vi "Perform_large_file_Analysis.vi"(0 "IntensityGraph in":refnum<vi>) -> (1 "Integral Spectrum":dbl[][](array[numeric]), 2 "size(s)":i32, 3 "Analysis_Data":T2, 4 "Spectrum Data":T1, 5 "Discr. Slope":cluster{"Array":dbl[], "Array":dbl[]})   [LabVIEW 2019]
uses:
  ESA_Data_Analysis_Global_VIs.vi
  <vilib>/Analysis/NI_AALPro.lvlib
panel:
  out "Ch#1 min peak index":i32
  out "Ch#2 min peak index":i32
  out "Ch#2 min peak":dbl
  out "Ch#1 min peak":dbl
  out "Waveform Graph":dbl[][](graph)
  out "Ch#2_Peak":dbl[](array[numeric])
  out "Ch#1_Peak":dbl[](array[numeric])
  out "channel name(s) out":string[](array[string])
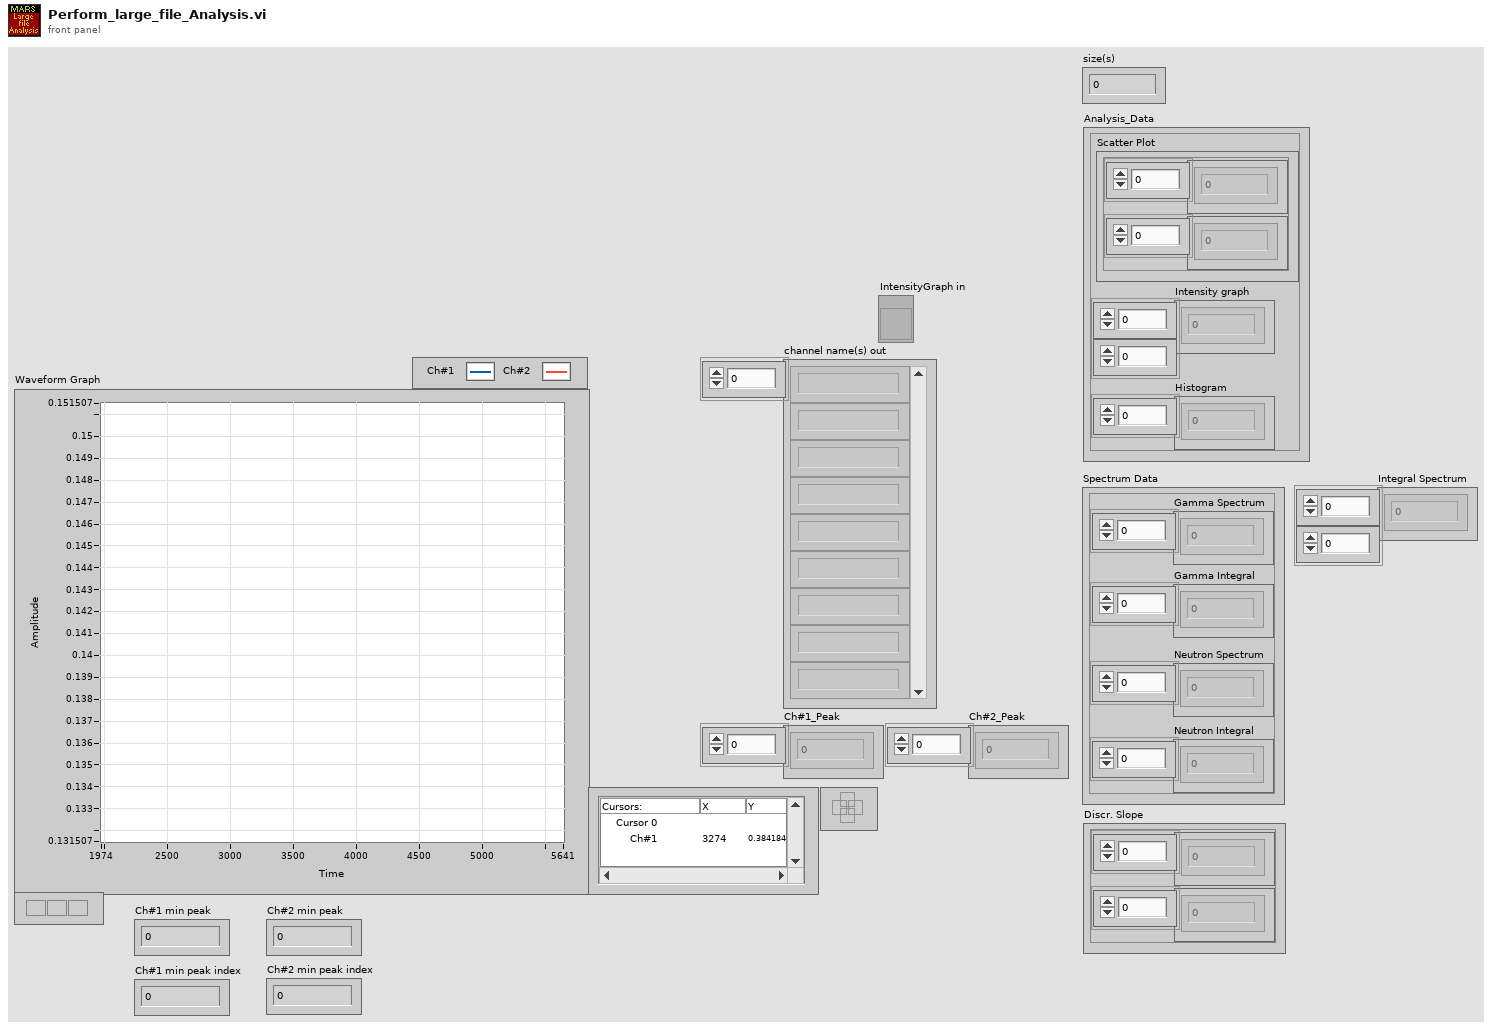
[diagram p1: front panel]
types:
  T1 = cluster{"Gamma Spectrum":dbl[], "Gamma Integral":dbl[], "Neutron Spectrum":dbl[], "Neutron Integral":dbl[]}
  T2 = cluster{"Scatter Plot":cluster{"Array":dbl[], "Array":dbl[]}, "Intensity graph":u32[][], "Histogram":u32[]}
  T3 = cluster{"Cursor.Cursor X1":dbl, "Cursor.Cursor Y1":dbl, "Cursor.Cursor X2":dbl, "Cursor.Cursor Y2":dbl}
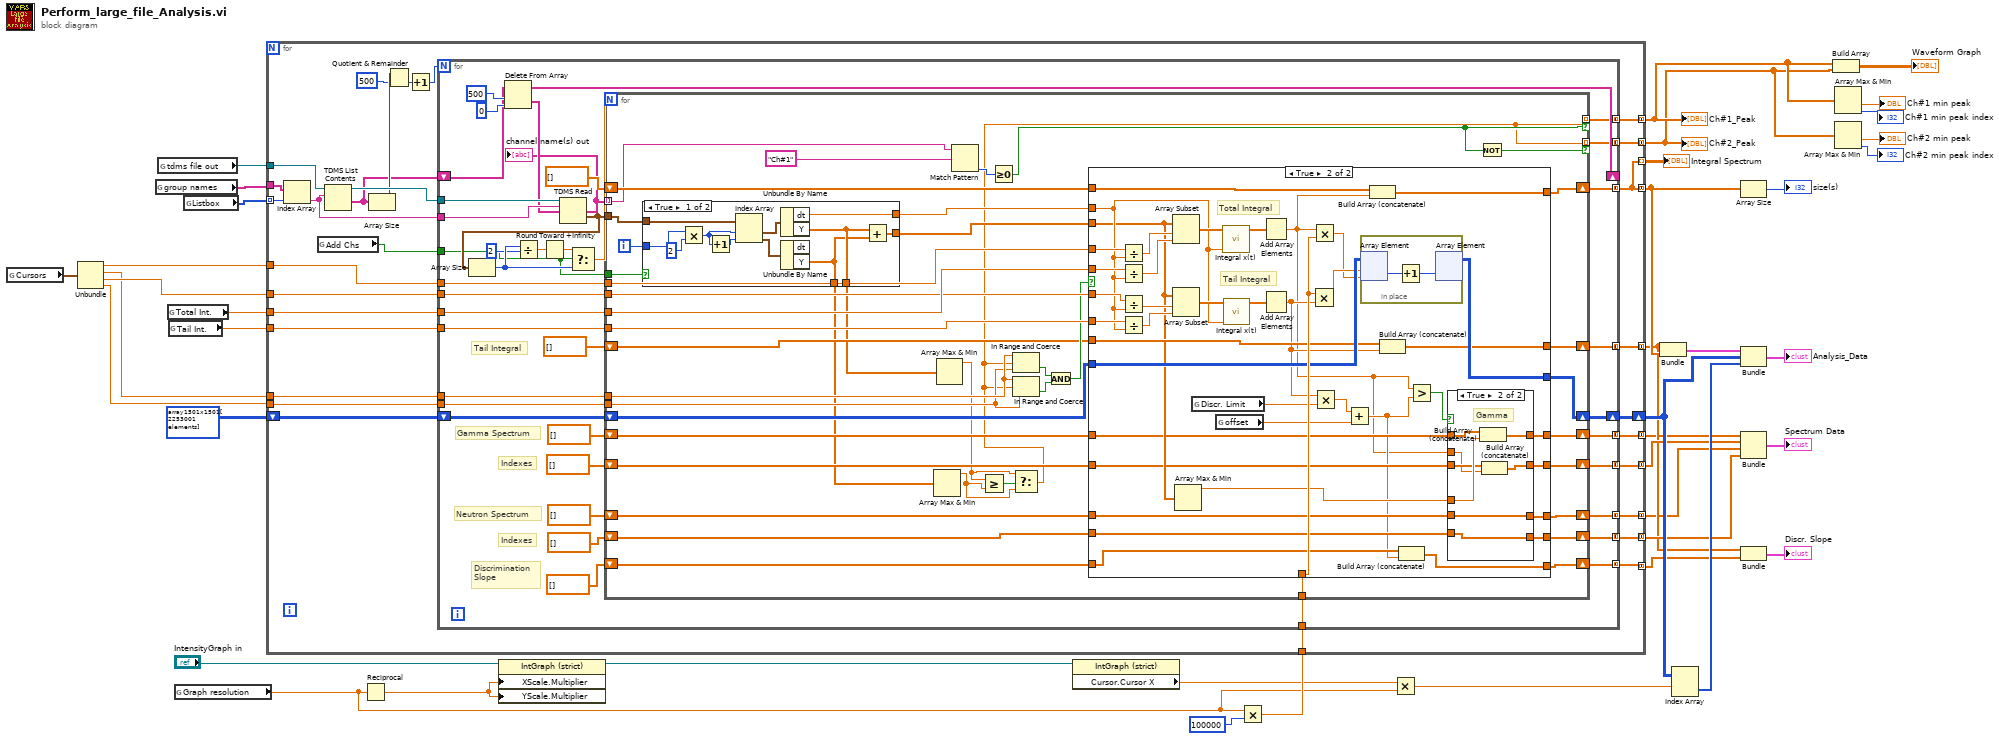
[diagram p0: block diagram]
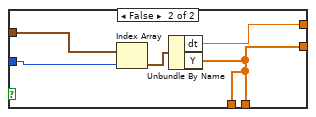
[diagram p2: hidden frame]
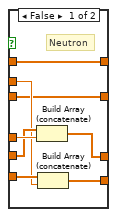
[diagram p4: hidden frame]
diagram:
  n1 = global read "ESA_Data_Analysis_Global_VIs.vi" "Cursors"() -> (w18:T3)
  n2 = Unbundle(w18) -> ("Cursor.Cursor X1"=w31:dbl, "Cursor.Cursor Y1"=w29:dbl, "Cursor.Cursor X2"=w30:dbl, "Cursor.Cursor Y2"=w28:dbl)
  n3 = global read "ESA_Data_Analysis_Global_VIs.vi" "group names"() -> (w20:string[])
  n4 = global read "ESA_Data_Analysis_Global_VIs.vi" "tdms file out"() -> (w21:refnum<k34>)
  n5 = global read "ESA_Data_Analysis_Global_VIs.vi" "Total Int."() -> (w24:dbl)
  n6 = global read "ESA_Data_Analysis_Global_VIs.vi" "Tail Int."() -> (w23:dbl)
  n7 = global read "ESA_Data_Analysis_Global_VIs.vi" "Graph resolution"() -> (w22:dbl)
  n8 = global read "ESA_Data_Analysis_Global_VIs.vi" "Listbox"() -> (w19:i32[])
  n9 = Reciprocal(x=w22) -> (1/x=w40:dbl)
  n10 = property on="Property Node" class="IntGraph (strict)"(reference="IntensityGraph in", "XScale.Multiplier"=w40, "YScale.Multiplier"=w40) -> (reference out=w36:refnum<vi>)  [unwired: 1 in, 1 out]
  n11 = property on="Property Node" class="IntGraph (strict)"(reference=w36) -> ("Cursor.Cursor X"=w35:dbl)  [unwired: 1 in, 2 out]
  n12 = Multiply(x=w22, y=100000) -> (x*y=w38:dbl)
  n13 = for {
    tunnel: w21 -> [w70]
    tunnel: w20 -> [w68]
    tunnel: w19 -> [w67] mode=indexing
    tunnel: w31 -> [w63]
    tunnel: w30 -> [w62]
    tunnel: w24 -> [w61]
    tunnel: w23 -> [w60]
    tunnel: w38 -> [w59]
    shift-right: [w57] -> w27
    shift-left: u32[][] array1501x1501[2253001 elements] -> [w58]
    tunnel: [w46] -> w33 mode=concatenating
    tunnel: [w56] -> w12 mode=concatenating
    tunnel: w29 -> [w53]
    tunnel: w28 -> [w52]
    tunnel: [w51] -> w9 mode=concatenating
    tunnel: [w50] -> w10 mode=concatenating
    tunnel: [w49] -> w17 mode=concatenating
    tunnel: [w48] -> w16 mode=concatenating
    tunnel: [w47] -> w13 mode=concatenating
    tunnel: [w46] -> w8 mode=indexing
    tunnel: [w44] -> w6 mode=concatenating
    tunnel: [w43] -> w5 mode=concatenating
    n14 = Index Array(array=w68, index=w67) -> (element=w64:string)
    n15 = global read "ESA_Data_Analysis_Global_VIs.vi" "Add Chs"() -> (w42:bool)
    n16 = TDMS List Contents(6:w64, 7:w70) -> (1:w55:string[], 3:w69:refnum<k34>)  [unwired: 1 in, 2 out]
    n17 = Array Size(array=w55) -> (size(s)=w66:i32)
    n18 = Quotient & Remainder(x=w66, y=500) -> (floor(x/y)=w54:i32)  [unwired: 1 out]
    n19 = Increment(x=w54) -> (x+1=w45:i32)
    n20 = for {
      N: w45 -> [_]
      tunnel: w69 -> [w110]
      tunnel: w64 -> [w100]
      tunnel: w63 -> [w109]
      tunnel: w62 -> [w108]
      tunnel: w61 -> [w107]
      tunnel: w60 -> [w106]
      tunnel: w59 -> [w105]
      shift-right: [w103] -> w57
      shift-left: w58 -> [w104]
      tunnel: [w102] -> w46 mode=concatenating
      tunnel: [w101] -> w56 mode=concatenating
      shift-right: [w96] -> _
      shift-left: w55 -> [w97]
      tunnel: w53 -> [w94]
      tunnel: w52 -> [w93]
      tunnel: [w88] -> w51 mode=concatenating
      tunnel: [w87] -> w50 mode=concatenating
      tunnel: [w85] -> w49 mode=concatenating
      tunnel: [w83] -> w48 mode=concatenating
      tunnel: [w81] -> w47 mode=concatenating
      tunnel: [w79] -> w44 mode=concatenating
      tunnel: [w78] -> w43 mode=concatenating
      tunnel: w42 -> [w71]
      # "Tail Integral"
      # "Discrimination\nSlope"
      # "Indexes"
      # "Indexes"
      # "Neutron Spectrum"
      # "Gamma Spectrum"
      n21 = Delete From Array(array=w97, length=500, index=0) -> (deleted portion=w95:string[], array with subset deleted=w96:string[])
      n22 = TDMS Read(0:w110, 5:w100, 7:w95) -> (8:w80:string[], 10:w77:waveform(dbl)[])  [unwired: 5 in, 4 out]
      "channel name(s) out" <- w80
      n23 = Array Size(array=w77) -> (size(s)=w76:i32)
      n24 = Divide(x=w76, y=2) -> (x/y=w73:dbl)
      n25 = Round Toward +Infinity(x=w73) -> (ceil(x): smallest int >= x=w72:dbl)
      n26 = Select(t=w72, s=w71, f=w76) -> (s? t:f=w74:dbl)
      n27 = for {
        N: w74 -> [_]
        tunnel: w77 -> [w120]
        tunnel: w109 -> [w152]
        tunnel: w107 -> [w151]
        tunnel: w108 -> [w150]
        tunnel: w106 -> [w149]
        tunnel: w105 -> [w147]
        shift-right: [w145] -> w103
        shift-left: w104 -> [w146]
        tunnel: w94 -> [w140]
        tunnel: w93 -> [w139]
        shift-right: [w121] -> w102
        shift-left: dbl[] [] -> [w138]
        shift-right: [w144] -> w101
        shift-left: dbl[] [] -> [w137]
        shift-right: [w135] -> w88
        shift-left: dbl[] [] -> [w136]
        shift-right: [w133] -> w87
        shift-left: dbl[] [] -> [w134]
        shift-right: [w131] -> w85
        shift-left: dbl[] [] -> [w132]
        shift-right: [w129] -> w83
        shift-left: dbl[] [] -> [w130]
        shift-right: [w127] -> w81
        shift-left: dbl[] [] -> [w128]
        tunnel: w80 -> [w125] mode=indexing
        tunnel: [w112] -> w79 mode=indexing if=w123
        tunnel: [w112] -> w78 mode=indexing if=w122
        tunnel: w71 -> [w111]
        i -> [w119]
        n28 = case shown="True" w111 {
          tunnel: [w163 w168] -> w148
          tunnel: w120 -> [w162 w167]
          tunnel: w119 -> [w160 w164]
          tunnel: [w155 w165] -> w118
          tunnel: [w154 w165] -> w117
          tunnel: [w153 w165] -> w116
          frame True {
            n29 = Multiply(x=w160, y=2) -> (x*y=w158:i32)
            n30 = Increment(x=w158) -> (x+1=w159:i32)
            n31 = Index Array(array=w162, index #1=w158, index #2=w159) -> (element #1=w161:waveform(dbl), element #2=w156:waveform(dbl))
            n32 = Unbundle By Name(w161) -> ("dt"=w163:dbl, "Y"=w155:dbl[])
            n33 = Unbundle By Name(w156) -> ("Y"=w153:dbl[])  [unwired: 1 out]
            n34 = Add(x=w155, y=w153) -> (x+y=w154:dbl[])
          }
          frame False {
            n35 = Index Array(array=w167, index=w164) -> (element=w166:waveform(dbl))
            n36 = Unbundle By Name(w166) -> ("dt"=w168:dbl, "Y"=w165:dbl[])
          }
        }
        n37 = Array Max & Min(array=w116) -> (max value=w113:dbl)  [unwired: 3 out]
        n38 = Array Max & Min(array=w118) -> (max value=w114:dbl)  [unwired: 3 out]
        n39 = Match Pattern(string=w125, regular expression="Ch#1") -> (offset past match=w124:i32)  [unwired: 1 in, 3 out]
        n40 = Greater Or Equal?(x=w114, y=w113) -> (x >= y?=w115:bool)
        n41 = Greater Or Equal To 0?(x=w124) -> (x >= 0?=w123:bool)
        n42 = Select(t=w114, s=w115, f=w113) -> (s? t:f=w112:dbl)
        n43 = In Range and Coerce(upper limit=w140, x=w112, lower limit=w139) -> (In Range?=w143:bool)  [unwired: 1 out]
        n44 = In Range and Coerce(upper limit=w140, x=w112, lower limit=w139) -> (In Range?=w142:bool)  [unwired: 1 out]
        n45 = And(x=w143, y=w142) -> (x .and. y?=w141:bool)
        n46 = case shown="True" w141 {
          tunnel: w152 -> [_ w213]
          tunnel: w151 -> [_ w212]
          tunnel: w150 -> [_ w211]
          tunnel: w149 -> [_ w210]
          tunnel: w117 -> [_ w197]
          tunnel: w148 -> [_ w205]
          tunnel: w147 -> [_ w204]
          tunnel: w146 -> [w174 w203]
          tunnel: [w174 w202] -> w145
          tunnel: [w176 w201] -> w121
          tunnel: [w175 w199] -> w144
          tunnel: w138 -> [w176 w200]
          tunnel: w137 -> [w175 w198]
          tunnel: w136 -> [w173 w194]
          tunnel: [w173 w193] -> w135
          tunnel: w134 -> [w172 w192]
          tunnel: [w172 w191] -> w133
          tunnel: w132 -> [w171 w189]
          tunnel: [w171 w188] -> w131
          tunnel: w130 -> [w170 w187]
          tunnel: [w170 w186] -> w129
          tunnel: w128 -> [w169 w182]
          tunnel: [w169 w181] -> w127
          frame False {
          }
          frame True {
            # "Total Integral"
            # "Tail Integral"
            n47 = Divide(x=w213, y=w205) -> (x/y=w217:dbl)
            n48 = Divide(x=w212, y=w205) -> (x/y=w216:dbl)
            n49 = Divide(x=w211, y=w205) -> (x/y=w214:dbl)
            n50 = Divide(x=w210, y=w205) -> (x/y=w215:dbl)
            n51 = Array Subset(array=w197, index=w217, length=w216) -> (w206:dbl[])
            n52 = Array Subset(array=w197, index=w214, length=w215) -> (w209:dbl[])
            n53 = Array Max & Min(array=w197) -> (max value=w195:dbl)  [unwired: 3 out]
            n54 = global read "ESA_Data_Analysis_Global_VIs.vi" "Discr. Limit"() -> (w190:dbl)
            n55 = global read "ESA_Data_Analysis_Global_VIs.vi" "offset"() -> (w183:dbl)
            n56 = call <vilib>:"Integral x(t).vi"("dt"=w205, "X"=w206) -> ("Integral X"=w208:dbl[])  [unwired: 8 in, 1 out]
            n57 = call <vilib>:"Integral x(t).vi"("dt"=w205, "X"=w209) -> ("Integral X"=w207:dbl[])  [unwired: 8 in, 1 out]
            n58 = Add Array Elements(numeric array=w208) -> (sum=w177:dbl)
            n59 = Add Array Elements(numeric array=w207) -> (sum=w179:dbl)
            n60 = Multiply(x=w204, y=w179) -> (x*y=w185:dbl)
            n61 = Multiply(x=w177, y=w204) -> (x*y=w178:dbl)
            n62 = Multiply(x=w179, y=w190) -> (x*y=w184:dbl)
            n63 = Add(x=w184, y=w183) -> (x+y=w180:dbl)
            n64 = in-place {
              n65 = in-place-array #1(w203, w185, w178) -> (w235:u32)
              n66 = Increment(x=w235) -> (x+1=w234:u32)
              n67 = in-place-array #1(w234) -> (w202:u32[][])  [unwired: 2 out]
            }
            n68 = Build Array (concatenate)(w200, w177) -> (w201:dbl[])
            n69 = Build Array (concatenate)(w198, w179) -> (w199:dbl[])
            n70 = Build Array (concatenate)(w182, w180) -> (w181:dbl[])
            n71 = Greater?(x=w177, y=w180) -> (0:w196:bool)
            n72 = case shown="True" w196 {
              tunnel: w195 -> [w225 w233]
              tunnel: [w223 w232] -> w193
              tunnel: w194 -> [w223 w231]
              tunnel: w192 -> [w224 w230]
              tunnel: [w222 w230] -> w191
              tunnel: w189 -> [w218 w229]
              tunnel: w177 -> [w220 w228]
              tunnel: [w218 w227] -> w188
              tunnel: w187 -> [w221 w226]
              tunnel: [w219 w226] -> w186
              frame False {
                # "Neutron"
                n73 = Build Array (concatenate)(w224, w225) -> (w222:dbl[])
                n74 = Build Array (concatenate)(w221, w220) -> (w219:dbl[])
              }
              frame True {
                # "Gamma"
                n75 = Build Array (concatenate)(w231, w233) -> (w232:dbl[])
                n76 = Build Array (concatenate)(w229, w228) -> (w227:dbl[])
              }
            }
          }
        }
        n77 = Not(x=w123) -> (.not. x?=w122:bool)
      }
    }
  }
  "Integral Spectrum" <- w8
  "Ch#1_Peak" <- w6
  "Ch#2_Peak" <- w5
  n78 = Multiply(x=w35, y=w22) -> (x*y=w41:dbl)
  n79 = Bundle(w12, w33) -> (w14:cluster{dbl[], dbl[]})  [unwired: 1 in]
  n80 = Index Array(array=w27, index (row)=w41) -> (element=w26:u32[])  [unwired: 1 in]
  n81 = Array Size(array=w33) -> (size(s)=→"size(s)":i32)
  n82 = Bundle(w14, w27, w26) -> (→"Analysis_Data":cluster{cluster{dbl[], dbl[]}, u32[][], u32[]})  [unwired: 1 in]
  n83 = Bundle(w9, w17, w10, w16) -> (→"Spectrum Data":cluster{dbl[], dbl[], dbl[], dbl[]})  [unwired: 1 in]
  n84 = Bundle(w12, w13) -> (→"Discr. Slope":cluster{dbl[], dbl[]})  [unwired: 1 in]
  n85 = Build Array(w6, w5) -> (→"Waveform Graph":dbl[][])
  n86 = Array Max & Min(array=w6) -> (min value=→"Ch#1 min peak":dbl, min index (indices)=→"Ch#1 min peak index":i32)  [unwired: 2 out]
  n87 = Array Max & Min(array=w5) -> (min value=→"Ch#2 min peak":dbl, min index (indices)=→"Ch#2 min peak index":i32)  [unwired: 2 out]
